vi "Create Threats table from Server DB.vi"(8 "error in":errorcluster) -> (0 "error out":errorcluster)   [LabVIEW 2010]
uses:
  <vilib>/addons/database/NI_Database_API.lvlib
  <vilib>/addons/database/Connection.llb/DB Tools Open Connec (Path).vi
  <vilib>/addons/database/Connection.llb/Conn Execute.vi
  <vilib>/addons/database/Recordset.llb/Rec Fetch Recordset Data (R).vi
  <vilib>/addons/database/Auxilliary.llb/DB Tools Cursor Type.ctl
  <vilib>/addons/database/Recordset.llb/Rec Destroy - Connection.vi
  <vilib>/addons/database/_DB Variant To Data/Database Variant To Data.xnode
  <vilib>/addons/database/Auxilliary.llb/DB Tools DataTypes.ctl
panel:
  in  "Table":string="Threats"
  out "column information":T2(array[cluster])
  out "columns":string[](array[string])
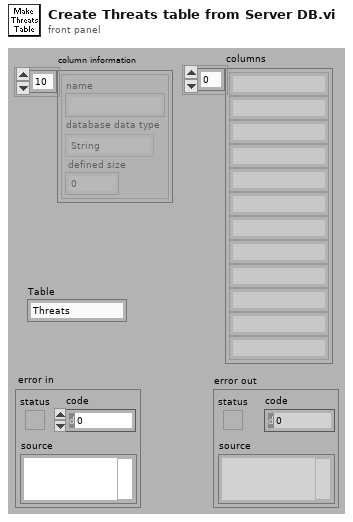
[diagram p1: front panel]
types:
  T1 = typedef "NI_Database_API.lvlib/DB Tools DataTypes.ctl" = enum16{"String", "Long (I32)", "Single (SGL)", "Double (DBL)", "Date/Time", "Binary"}
  T2 = cluster{"name":string, "database data type":T1, "defined size":i32}[]
  T3 = typedef "NI_Database_API.lvlib/DB Tools Cursor Type.ctl" = enum16{"forward-only", "keyset", "dynamic", "static"}
  T4 = typedef "NI_Database_API.lvlib/Conn ObjectReference.ctl" = refnum<k1>
  T5 = typedef "NI_Database_API.lvlib/Rec ObjectReference.ctl" = refnum<k1>
  T6 = cluster{"data":i32, "data":i32, "data":i32, "trimmed string":string, "trimmed string":string, "data":i32, "data":sgl, "data":i32, "data":i32, "data":i32, "trimmed string":string}
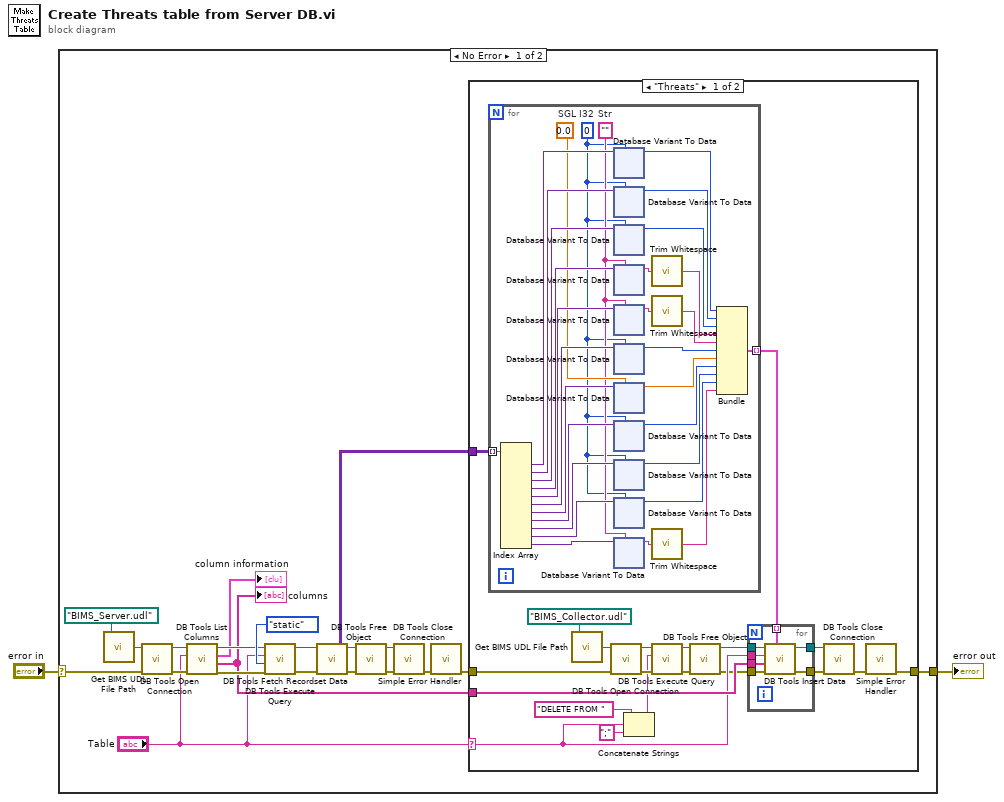
[diagram p0: block diagram]
diagram:
  n1 = case shown="No Error" "error in" {
    selector: "error in" -> [w3 w434]
    tunnel: [w4 w434] -> w2
    frame No Error {
      n2 = call "Get BIMS UDL File Path.vi"("UDL file name"=path "BIMS_Server.udl") -> ("Full UDL file path"=w22:path)
      n3 = call-poly <vilib>:"DB Tools Open Connection.vi"("error in (no error)"=w3, "connection information"=w22) -> ("error out"=w20:errorcluster, "connection reference"=w21:T4)  [unwired: 3 in, 3 out]
      n4 = call <vilib>:"DB Tools List Columns.vi"("error in (no error)"=w20, "table"="Table", "connection reference"=w21) -> ("error out"=w9:errorcluster, "columns"=w6:string[], "column information"=→"column information":T2, "connection reference out"=w10:T4)  [unwired: 1 out]
      "columns" <- w6
      n5 = call-poly <vilib>:"DB Tools Execute Query.vi"("error in (no error)"=w9, "cursor type"=DB_Tools_Cursor_Type."static", "SQL query"="Table", "connection reference"=w10) -> ("error out"=w13:errorcluster, "recordset reference"=w14:T5)  [unwired: 4 out]
      n6 = call-poly <vilib>:"DB Tools Fetch Recordset Data.vi"("error in (no error)"=w13, "recordset reference"=w14) -> ("error out"=w16:errorcluster, "recordset data"=w11:variant[][], "recordset reference out"=w15:T5)  [unwired: 3 out]
      n7 = call-poly <vilib>:"DB Tools Free Object.vi"("error in (no error)"=w16, "recordset reference"=w15) -> ("error out"=w18:errorcluster, "connection reference"=w17:T4)  [unwired: 8 out]
      n8 = call <vilib>:"DB Tools Close Connection.vi"("error in (no error)"=w18, "connection reference"=w17) -> ("error out"=w8:errorcluster)  [unwired: 5 out]
      n9 = call <vilib>:"Simple Error Handler.vi"("error in (no error)"=w8) -> ("error out"=w19:errorcluster)  [unwired: 1 in, 7 out]
      n10 = case shown="\"Threats\"" "Table" {
        selector: "Table" -> [w30 _]
        tunnel: w19 -> [w43 w433]
        tunnel: w11 -> [w42 _]
        tunnel: w6 -> [w38 _]
        tunnel: [w34 w433] -> w4
        frame "Threats" {
          n11 = for {
            tunnel: [w59] -> w35 mode=indexing
            tunnel: w42 -> [w80] mode=indexing
            w66 = sgl 0.0  # SGL
            w61 = ""  # Str
            w57 = 0  # I32
            n12 = Index Array(array=w80) -> (element #1=w79:variant, element #2=w78:variant, element #3=w75:variant, element #4=w74:variant, element #5=w73:variant, element #6=w72:variant, element #7=w71:variant, element #8=w70:variant, element #9=w65:variant, element #10=w63:variant, element #11=w60:variant)  [unwired: 11 in]
            n13 = xnode ("Database Variant To Data")("database variant"=w79, "type"=w57) -> ("data"=w58:i32)  [unwired: 1 in, 1 out]
            n14 = xnode "Database Variant To Data"("database variant"=w78, "type"=w57) -> ("data"=w77:i32)  [unwired: 1 in, 1 out]
            n15 = xnode "Database Variant To Data"("database variant"=w75, "type"=w57) -> ("data"=w76:i32)  [unwired: 1 in, 1 out]
            n16 = xnode "Database Variant To Data"("database variant"=w74, "type"=w61) -> ("data"=w56:string)  [unwired: 1 in, 1 out]
            n17 = xnode ("Database Variant To Data")("database variant"=w73, "type"=w61) -> ("data"=w54:string)  [unwired: 1 in, 1 out]
            n18 = xnode "Database Variant To Data"("database variant"=w72, "type"=w57) -> ("data"=w69:i32)  [unwired: 1 in, 1 out]
            n19 = xnode "Database Variant To Data"("database variant"=w71, "type"=w66) -> ("data"=w68:sgl)  [unwired: 1 in, 1 out]
            n20 = xnode "Database Variant To Data"("database variant"=w70, "type"=w57) -> ("data"=w67:i32)  [unwired: 1 in, 1 out]
            n21 = xnode "Database Variant To Data"("database variant"=w65, "type"=w57) -> ("data"=w64:i32)  [unwired: 1 in, 1 out]
            n22 = xnode "Database Variant To Data"("database variant"=w63, "type"=w57) -> ("data"=w62:i32)  [unwired: 1 in, 1 out]
            n23 = xnode "Database Variant To Data"("database variant"=w60, "type"=w61) -> ("data"=w52:string)  [unwired: 1 in, 1 out]
            n24 = call <vilib>:"Trim Whitespace.vi"("string"=w56) -> ("trimmed string"=w55:string)  [unwired: 1 in]
            n25 = call <vilib>:"Trim Whitespace.vi"("string"=w54) -> ("trimmed string"=w53:string)  [unwired: 1 in]
            n26 = call <vilib>:"Trim Whitespace.vi"("string"=w52) -> ("trimmed string"=w51:string)  [unwired: 1 in]
            n27 = Bundle("data"=w58, "data"=w77, "data"=w76, "trimmed string"=w55, "trimmed string"=w53, "data"=w69, "data"=w68, "data"=w67, "data"=w64, "data"=w62, "trimmed string"=w51) -> (w59:T6)  [unwired: 1 out]
          }
          n28 = call "Get BIMS UDL File Path.vi"("UDL file name"=path "BIMS_Collector.udl") -> ("Full UDL file path"=w41:path)
          n29 = call-poly <vilib>:"DB Tools Open Connection.vi"("error in (no error)"=w43, "connection information"=w41) -> ("error out"=w33:errorcluster, "connection reference"=w29:T4)  [unwired: 3 in, 3 out]
          n30 = Concatenate Strings("DELETE FROM " ("SQL query"), w30, ";" ("string")) -> (w31:string)
          n31 = call-poly <vilib>:"DB Tools Execute Query.vi"("error in (no error)"=w33, "SQL query"=w31, "connection reference"=w29) -> ("error out"=w27:errorcluster, "recordset reference"=w25:T5)  [unwired: 1 in, 4 out]
          n32 = call-poly <vilib>:"DB Tools Free Object.vi"("error in (no error)"=w27, "recordset reference"=w25) -> ("error out"=w26:errorcluster, "connection reference"=w24:T4)  [unwired: 8 out]
          n33 = for {
            tunnel: [w50] -> w36
            tunnel: [w46] -> w37
            tunnel: w26 -> [w49]
            tunnel: w30 -> [w48]
            tunnel: w35 -> [w45] mode=indexing
            tunnel: w38 -> [w47]
            tunnel: w24 -> [w44]
            n34 = call <vilib>:"DB Tools Insert Data.vi"("data"=w45, "error in (no error)"=w49, "columns"=w47, "table"=w48, "connection reference"=w44) -> ("error out"=w46:errorcluster, "connection reference out"=w50:T4)  [unwired: 2 in, 3 out]
          }
          n35 = call <vilib>:"DB Tools Close Connection.vi"("error in (no error)"=w37, "connection reference"=w36) -> ("error out"=w40:errorcluster)  [unwired: 5 out]
          n36 = call <vilib>:"Simple Error Handler.vi"("error in (no error)"=w40) -> ("error out"=w34:errorcluster)  [unwired: 1 in, 7 out]
        }
        frame "Information", Default {
          # "The following case has a structure determined for \n  the Threats table in the BIMS server.\n\n  The data retieved from the table is site specific."
        }
      }
    }
    frame Error {
    }
  }
  "error out" <- w2
